vi "Search 2D Array for Sub Array.vi"(9 "Search Column":i32, 10 "Search Value":string, 11 "Raw Table":string[][](array[string])) -> (3 "Search Result":string[][](array[string]))   [LabVIEW 2010]
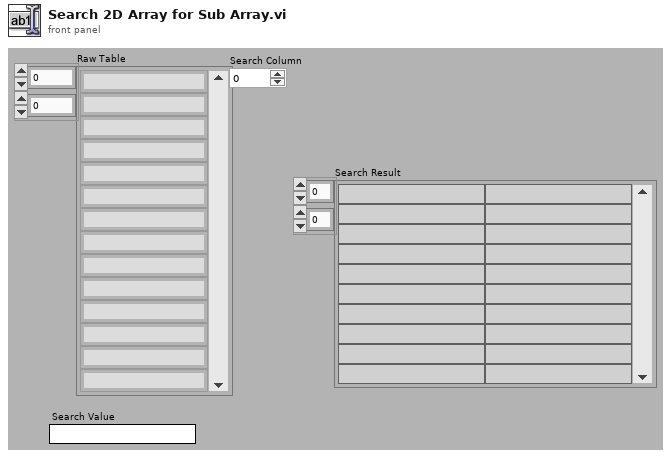
[diagram p1: front panel]
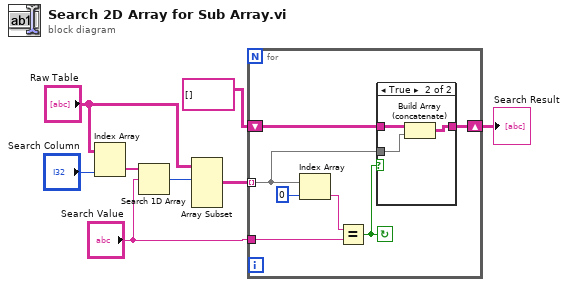
[diagram p0: block diagram]
diagram:
  n1 = Index Array(array="Raw Table", index (col)="Search Column") -> (element=w7:string[])  [unwired: 1 in]
  n2 = Search 1D Array(1D array=w7, element="Search Value") -> (index of element=w5:i32)  [unwired: 1 in]
  n3 = Array Subset(array="Raw Table", index (row)=w5) -> (w4:string[][])  [unwired: 3 in]
  n4 = for {
    tunnel: w4 -> [w12] mode=indexing
    tunnel: "Search Value" -> [w13]
    shift-right: [w11] -> w3
    shift-left: string[][] [] -> [w10]
    stop <- w9 continue-if-true
    n5 = Index Array(array=w12, index=0) -> (element=w14:string)
    n6 = Equal?(x=w14, y=w13) -> (x = y?=w9:bool)
    n7 = case shown="True" w9 {
      tunnel: w12 -> [_ w19]
      tunnel: [w16 w18] -> w11
      tunnel: w10 -> [w16 w17]
      frame False {
      }
      frame True {
        n8 = Build Array (concatenate)(w17, w19) -> (w18:string[][])
      }
    }
  }
  "Search Result" <- w3
